vi "MS Operation Thorlabs.vi"(6 "OCT Z PID Gains":cluster{"Kp":dbl, "Kd":dbl, "Ki":dbl}={"Kp"=0.0003, "Kd"=0.0001, "Ki"=0.01}, 8 "error in":errorcluster, 9 "OCT Prev Posit":dbl, 11 "FPGA VI Reference In":refnum<k20>) -> (0 "error out":errorcluster, 1 "OCT Last Posit":dbl, 3 "FPGA VI Reference Out":refnum<k20>)   [LabVIEW 2016]
uses:
  Subsystems/Global Variables.vi
  <vilib>/Platform/TimedLoop/XDataNode/wakeup.ctl
  <vilib>/Platform/TimedLoop/XDataNode/XDNodeRunTimeDep.lvlib
  <vilib>/Platform/TimedLoop/XDataNode/nitl_modes.ctl
  <vilib>/Platform/TimedLoop/XDataNode/timing_clust.ctl
  <vilib>/platform/TimedLoop/XDataNode/XDataNode.xnode
  <vilib>/rvi/interface/nirviReadWriteControl/nirviReadWriteControl.xnode
  Library/KevinLibraryAll/labview/KevLib01.lvlib
  FPGA Bitfiles/PhantomControlPI_FPGATarget_QuadCtr2_E2412E44.lvbitx
  IRISS_FPGA_IO.vi
  NiFpgaLv.dll
  <vilib>/Utility/error.llb/Error Cluster From Error Code.vi
  <vilib>/rvi/errors/niLvFpgaAdjustHostInterfaceError.vi
panel:
  out "Free":dbl[](array[numeric])
  out "Rigid":dbl[](array[numeric])
  out "Hydration On/Off":bool
  out "vac cmd":dbl
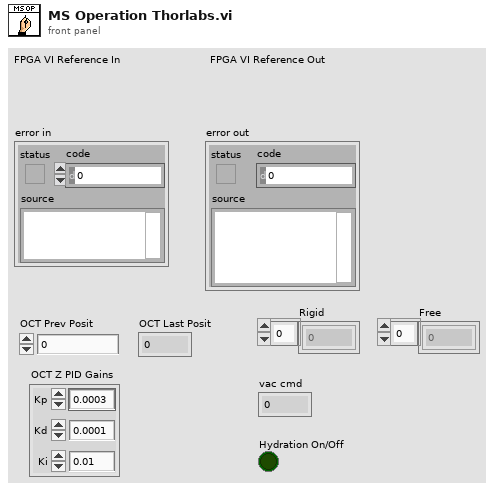
[diagram p1: front panel]
types:
  T1 = typedef "XDNodeRunTimeDep.lvlib/timing_clust.ctl" = cluster{"Expected End [f-1]":u64, "Actual End [f-1]":u64, "Finished Late? [f-1]":bool, "Expected End [i-1]":u64, "Actual End [i-1]":u64, "Finished Late? [i-1]":bool, "Expected Start [i]":u64, "Actual Start [i]":u64, "Expected Start [f]":u64, "Actual Start [f]":u64, "Source Name":string, "Structure Name":string, "Period":i64, "Deadline":i64, "Offset":i64, "Start":i64, "Priority":i32, "Timeout":i32, "Mode":T2, "Wakeup Reason":T3, "Error":errorcluster, "Source Type":string, "Secondary Source Type":string, "Global End Time":u64, "Global Start Time":u64, "Frame Duration":u64, "Iteration Duration":u64, "Assigned CPU":i32, "I/O Scan Engine Mode":u32}
  T2 = typedef "XDNodeRunTimeDep.lvlib/nitl_modes.ctl" = enum32{"No Change", "Process missed periods, maintain original phase", "Discard missed periods, maintain original phase", "Process missed periods, ignore original phase", "Discard missed periods, ignore original phase"}
  T3 = typedef "XDNodeRunTimeDep.lvlib/wakeup.ctl" = enum32{"Normal", "Aborted", "Asynchronous wakeup", "Timing source error", "Timed loop error", "Timeout"}
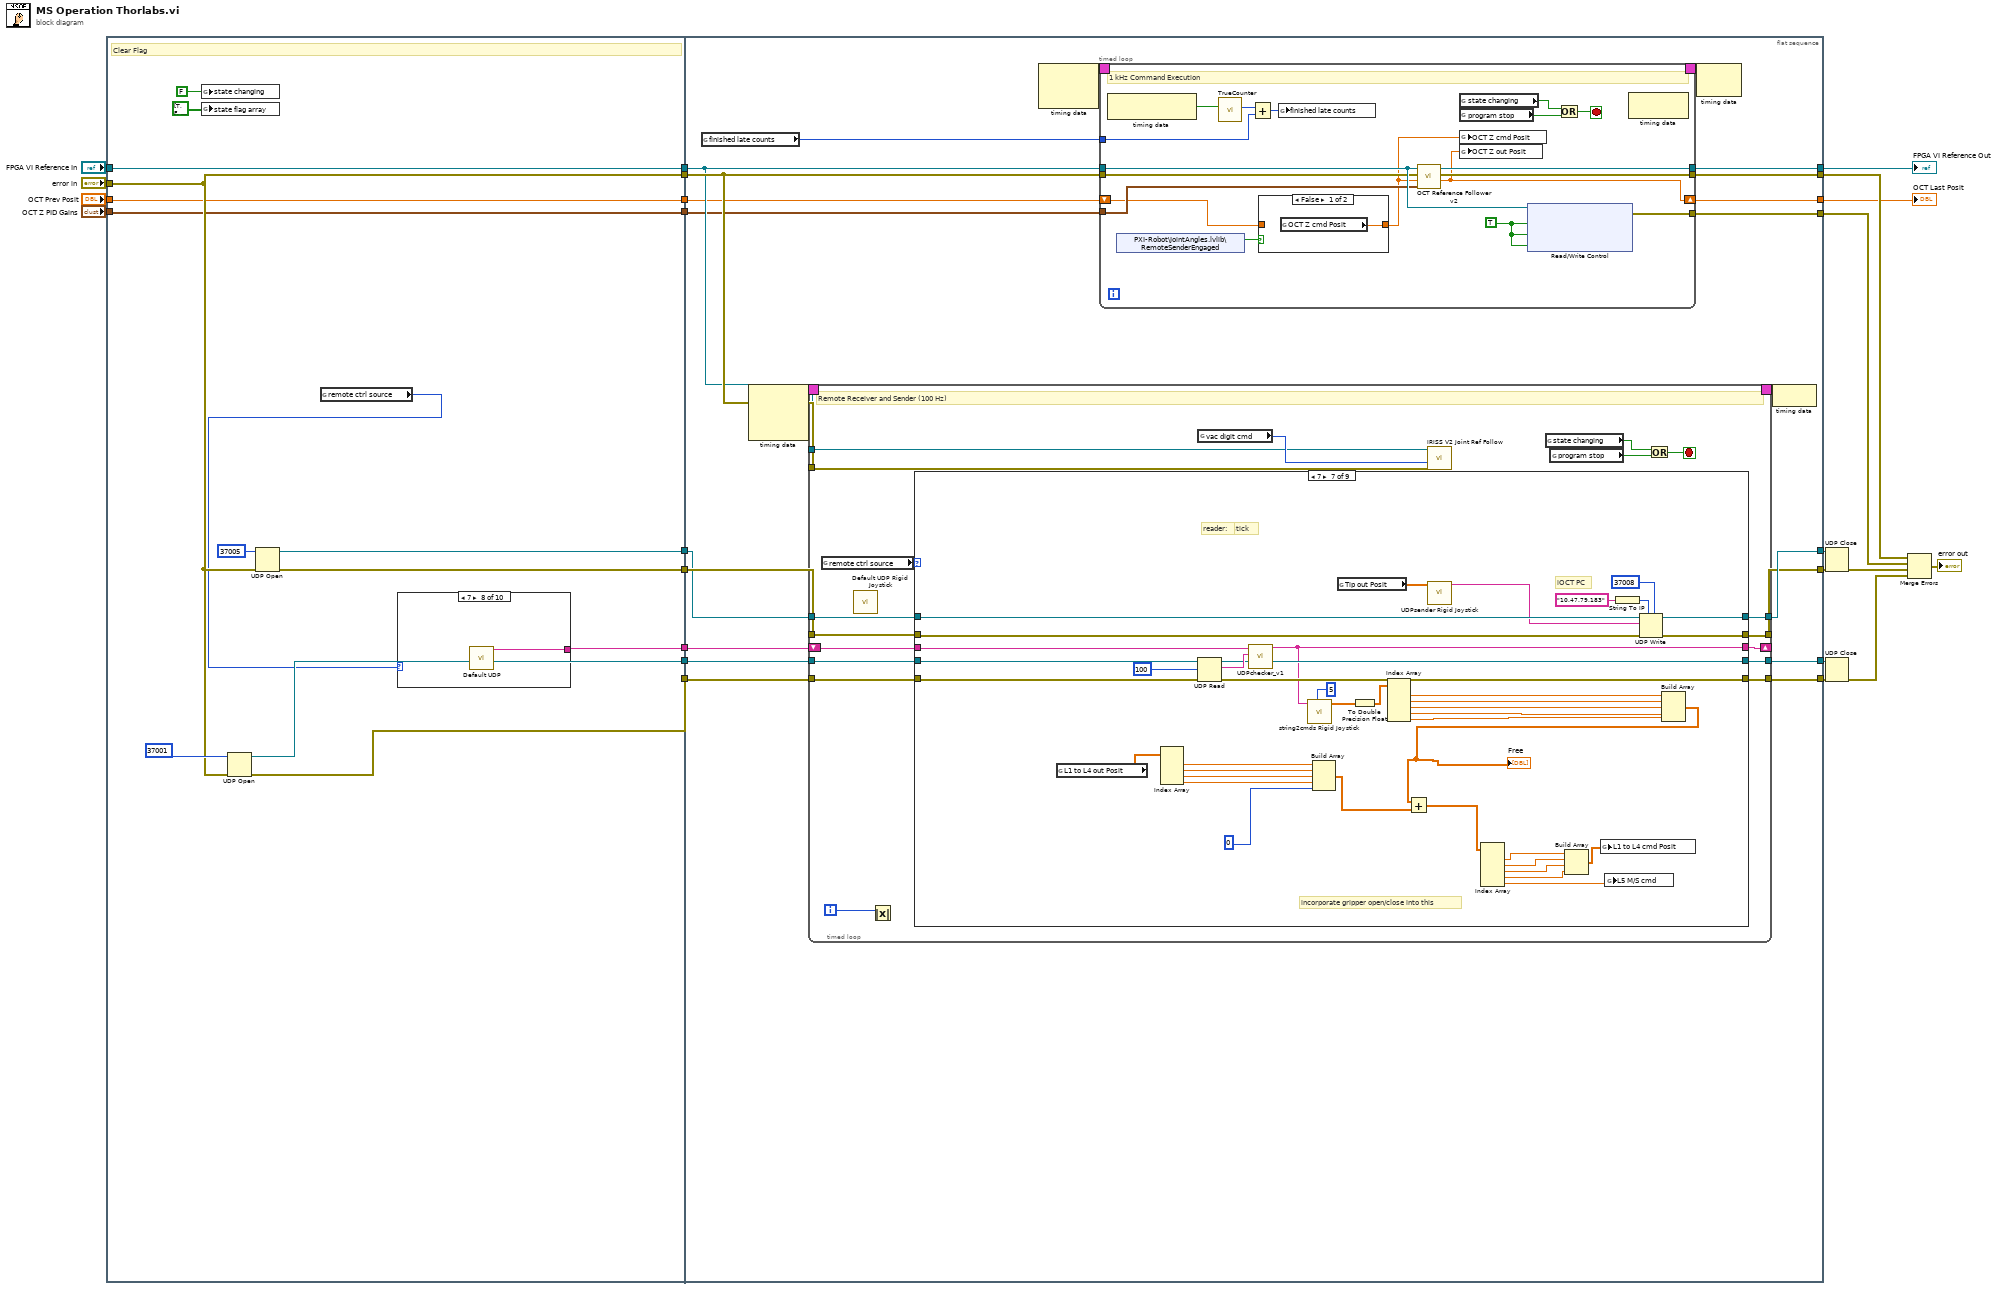
[diagram p0: block diagram]
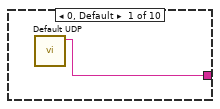
[diagram p2: hidden frame]
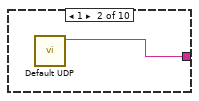
[diagram p3: hidden frame]
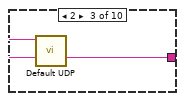
[diagram p4: hidden frame]
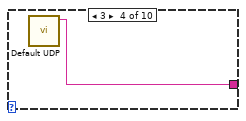
[diagram p5: hidden frame]
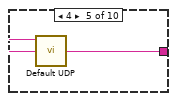
[diagram p6: hidden frame]
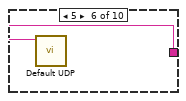
[diagram p7: hidden frame]
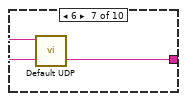
[diagram p8: hidden frame]
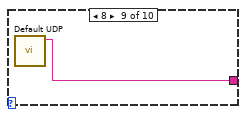
[diagram p9: hidden frame]
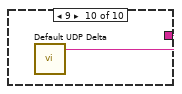
[diagram p10: hidden frame]
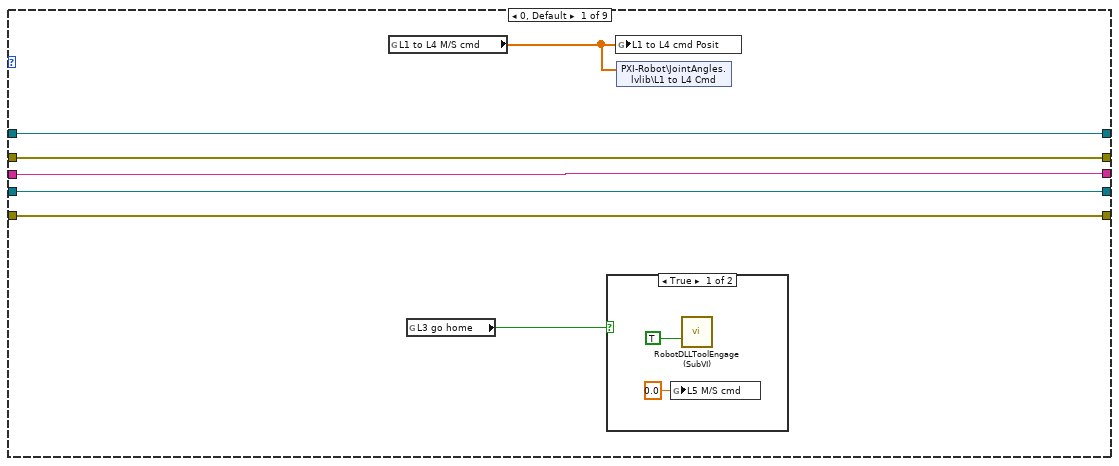
[diagram p11: hidden frame]
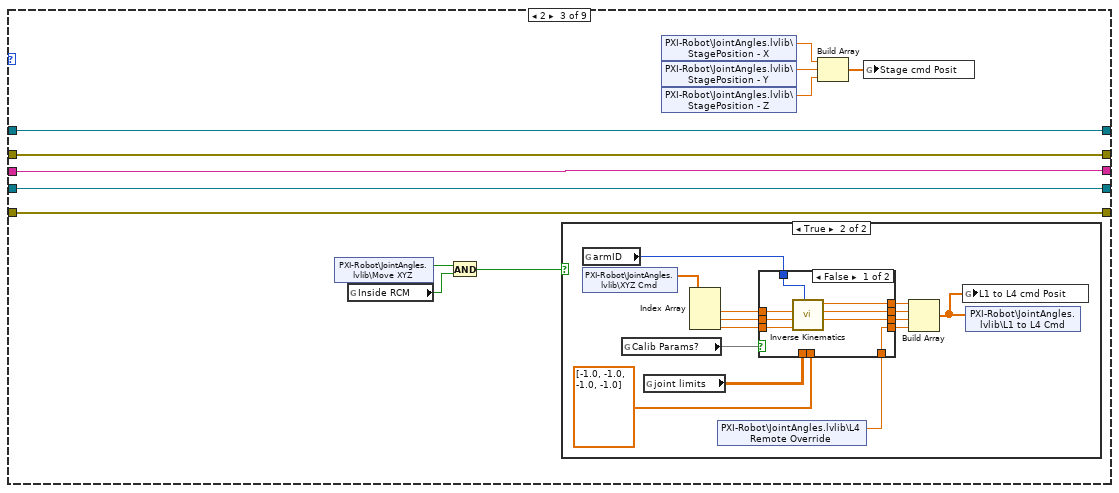
[diagram p14: hidden frame]
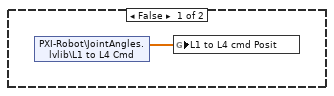
[diagram p15: hidden frame]
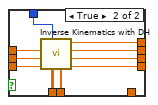
[diagram p16: hidden frame]
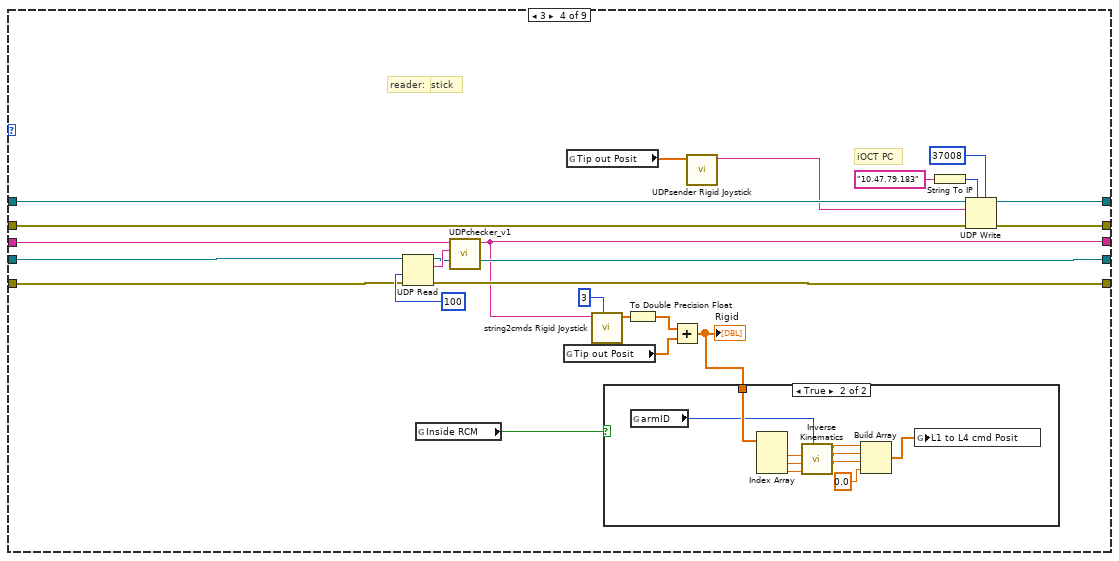
[diagram p17: hidden frame]
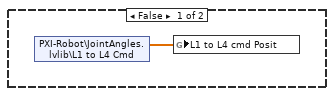
[diagram p18: hidden frame]
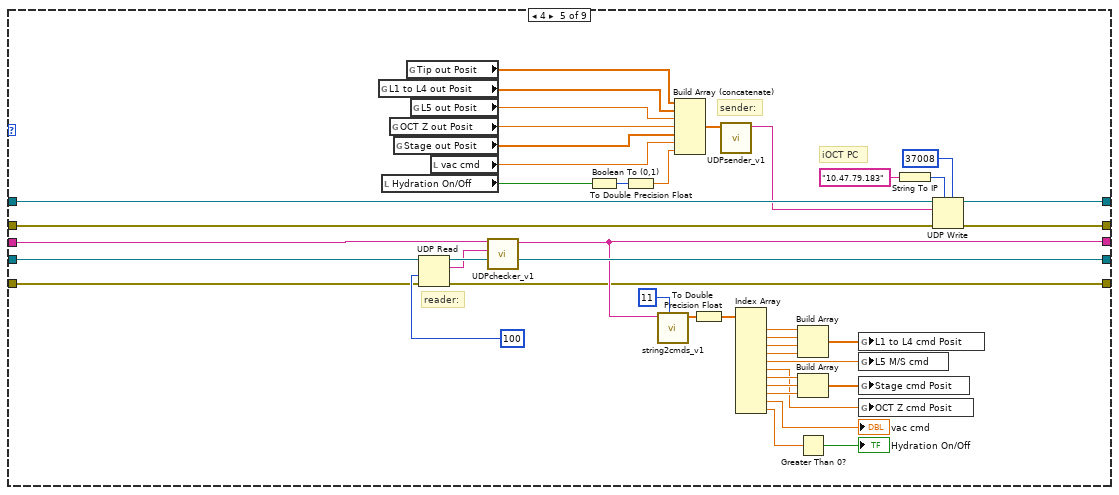
[diagram p19: hidden frame]
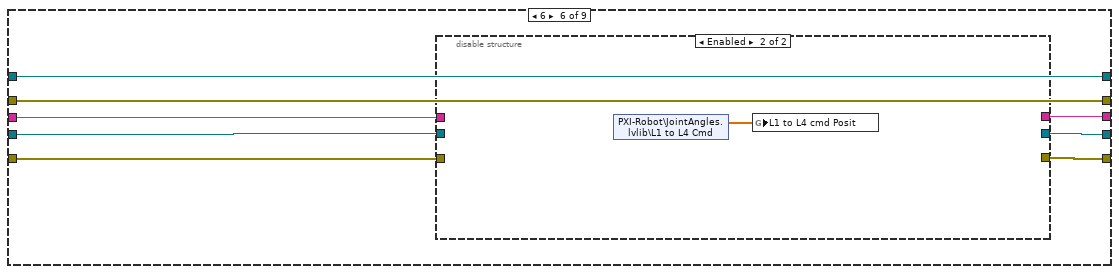
[diagram p20: hidden frame]
diagram:
  n1 = flat-sequence {
    tunnel: [w36] -> w24
    tunnel: "FPGA VI Reference In" -> [w36]
    tunnel: [w28] -> w22
    tunnel: "error in" -> [w28]
    tunnel: [w29] -> w20
    tunnel: [w33] -> w18
    tunnel: [w32] -> w17
    tunnel: [w31] -> w16
    tunnel: [w30] -> w15
    tunnel: [w27] -> w5
    tunnel: "OCT Prev Posit" -> [w27]
    tunnel: [w26] -> w3
    tunnel: "OCT Z PID Gains" -> [w26]
    tunnel: w24 -> [w52]
    tunnel: w22 -> [w53]
    tunnel: [w68] -> w6
    tunnel: [w67] -> w7
    tunnel: [w65] -> w21
    tunnel: w20 -> [w58]
    tunnel: w18 -> [w62]
    tunnel: w17 -> [w61]
    tunnel: w16 -> [w60]
    tunnel: w15 -> [w59]
    tunnel: [w57] -> w12
    tunnel: [w56] -> w11
    tunnel: [w55] -> w10
    tunnel: [w54] -> w9
    tunnel: w5 -> [w51]
    tunnel: w3 -> [w50]
    tunnel: [w49] -> w1
    frame #0 {
      # "Clear Flag"
      n2 = global write "Global Variables.vi" "state changing"(FALSE ("state changing")) -> ()
      n3 = global write "Global Variables.vi" "state flag array"(bool[] [TRUE, FALSE, FALSE, FALSE, FALSE, FALSE, FALSE, FALSE, FALSE] ("state flag array")) -> ()
      n4 = UDP Open(8:w28, 11:u16 37001 ("port")) -> (port=w31:refnum<k16>, 0:w30:errorcluster)  [unwired: 3 in, 1 out]
      n5 = UDP Open(8:w28, 11:u16 37005 ("port")) -> (port=w32:refnum<k16>, 0:w33:errorcluster)  [unwired: 3 in, 1 out]
      n6 = global read "Global Variables.vi" "remote ctrl source"() -> (w25:u16)
      n7 = case shown="7" w25 {
        tunnel: [w39 w40 w41 w42 w43 w44 w45 w46 w47 w48] -> w29
        frame 0, Default {
          n8 = call "Default UDP.vi"() -> ("String"=w39:string)  [unwired: 11 in]
        }
        frame 1 {
          n9 = call "Default UDP.vi"() -> ("String"=w40:string)  [unwired: 11 in]
        }
        frame 2 {
          n10 = call "Default UDP.vi"() -> ("String"=w41:string)  [unwired: 11 in]
        }
        frame 3 {
          n11 = call "Default UDP.vi"() -> ("String"=w42:string)  [unwired: 11 in]
        }
        frame 4 {
          n12 = call "Default UDP.vi"() -> ("String"=w43:string)  [unwired: 11 in]
        }
        frame 5 {
          n13 = call "Default UDP.vi"() -> ("String"=w44:string)  [unwired: 11 in]
        }
        frame 6 {
          n14 = call "Default UDP.vi"() -> ("String"=w45:string)  [unwired: 11 in]
        }
        frame 7 {
          n15 = call "Default UDP.vi"() -> ("String"=w46:string)  [unwired: 11 in]
        }
        frame 8 {
          n16 = call "Default UDP.vi"() -> ("String"=w47:string)  [unwired: 11 in]
        }
        frame 9 {
          n17 = call "Default UDP Delta.vi"() -> ("String"=w48:string)  [unwired: 11 in]
        }
      }
    }
    frame #1 {
      n18 = global read "Global Variables.vi" "finished late counts"() -> (w66:u16)
      n19 = node-c288() -> (w64:T1)  [unwired: 3 in]
      n20 = timed-loop {
        timing: w64 -> [_]
        timing-out: [_] -> w63
        tunnel: w60 -> [w88]
        tunnel: [w87] -> w55
        shift-right: [w85] -> _
        shift-left: w58 -> [w86]
        tunnel: w61 -> [w84]
        tunnel: w62 -> [w83]
        tunnel: [w82] -> w57
        tunnel: [w81] -> w56
        tunnel: w59 -> [w80]
        tunnel: [w79] -> w54
        tunnel: w52 -> [w73]
        tunnel: w53 -> [w72]
        i -> [w71]
        stop <- w76 stop-if-true
        # "Remote Receiver and Sender (100 Hz)"
        n21 = global read "Global Variables.vi" "remote ctrl source"() -> (w75:u16)
        n22 = call "Default UDP Rigid Joystick.vi"() -> ()  [unwired: 11 in, 1 out]
        n23 = Absolute Value(x=w71) -> ()  [unwired: 1 out]
        n24 = case shown="7" w75 {
          tunnel: w88 -> [w92 w99 w111 w168 w223 w229 w287 w292 w318]
          tunnel: [w92 w99 w111 w164 w222 w230 w285 w292 w319] -> w87
          tunnel: w86 -> [w93 w100 w112 w162 w182 w232 w283 w293 w325]
          tunnel: [w93 w100 w112 w161 w209 w231 w282 w293 w314] -> w85
          tunnel: w84 -> [w95 w102 w114 w155 w207 w225 w278 w311 w326]
          tunnel: w83 -> [w94 w101 w113 w153 w206 w226 w276 w310 w324]
          tunnel: [w95 w102 w114 w154 w202 w225 w277 w306 w320] -> w82
          tunnel: [w94 w101 w113 w152 w201 w226 w275 w305 w323] -> w81
          tunnel: w80 -> [w91 w98 w110 w167 w200 w227 w286 w291 w322]
          tunnel: [w91 w98 w110 w163 w199 w228 w284 w291 w321] -> w79
          frame 0, Default {
            n25 = global read "Global Variables.vi" "L1 to L4 M/S cmd"() -> (w89:dbl[])
            n26 = global read "Global Variables.vi" "L3 go home"() -> (w90:bool)
            n27 = case shown="True" w90 {
              frame True {
                n28 = global write "Global Variables.vi" "L5 M/S cmd"(0.0 ("L5 M/S cmd")) -> ()
                n29 = call "RobotDLLToolEngage (SubVI).vi"("Tool Fast Retraction"=TRUE ("Tool Withdraw")) -> ()  [unwired: 18 in, 1 out]
              }
              frame False {
              }
            }
            n30 = global write "Global Variables.vi" "L1 to L4 cmd Posit"(w89) -> ()
            n31 = shared-variable "PXI-Robot\\JointAngles.lvlib\\L1 to L4 Cmd"(w89) -> ()  [unwired: 1 in, 1 out]
          }
          frame 1 {
          }
          frame 2 {
            n32 = shared-variable "PXI-Robot\\JointAngles.lvlib\\Move XYZ"() -> (w108:bool)  [unwired: 1 in, 1 out]
            n33 = global read "Global Variables.vi" "Inside RCM"() -> (w107:bool)
            n34 = And(x=w108, y=w107) -> (x .and. y?=w109:bool)
            n35 = case shown="True" w109 {
              frame False {
                n36 = shared-variable "PXI-Robot\\JointAngles.lvlib\\L1 to L4 Cmd"() -> (w115:dbl[])  [unwired: 1 in, 1 out]
                n37 = global write "Global Variables.vi" "L1 to L4 cmd Posit"(w115) -> ()
              }
              frame True {
                n38 = global read "Global Variables.vi" "armID"() -> (w127:i32)
                n39 = shared-variable "PXI-Robot\\JointAngles.lvlib\\XYZ Cmd"() -> (w129:dbl[])  [unwired: 1 in, 1 out]
                n40 = global read "Global Variables.vi" "Calib Params?"() -> (w116)
                n41 = global read "Global Variables.vi" "joint limits"() -> (w119:dbl[][])
                n42 = Index Array(array=w129) -> (element #1=w126:dbl, element #2=w125:dbl, element #3=w124:dbl)  [unwired: 3 in]
                n43 = shared-variable "PXI-Robot\\JointAngles.lvlib\\L4 Remote Override"() -> (w117:dbl)  [unwired: 1 in, 1 out]
                n44 = case shown="False" w116 {
                  tunnel: w127 -> [w130 w147]
                  tunnel: w126 -> [w137 w146]
                  tunnel: w125 -> [w136 w145]
                  tunnel: w124 -> [w135 w144]
                  tunnel: [w134 w143] -> w123
                  tunnel: [w133 w142] -> w122
                  tunnel: [w132 w141] -> w121
                  tunnel: dbl[] [-1.0, -1.0, -1.0, -1.0] ("Initial guess") -> [_ w140]
                  tunnel: w119 -> [_ w139]
                  tunnel: [w131 w138] -> w118
                  tunnel: w117 -> [w131 _]
                  frame False {
                    n45 = call "Inverse Kinematics.vi"("armID"=w130, "z"=w135, "y"=w136, "x"=w137) -> ("j3"=w132:dbl, "j2"=w133:dbl, "j1"=w134:dbl)  [unwired: 4 in, 1 out]
                  }
                  frame True {
                    n46 = call "Inverse Kinematics with DH.vi"("Initial guess"=w140, "Joint Limits"=w139, "armID"=w147, "z"=w144, "y"=w145, "x"=w146) -> ("j4"=w138:dbl, "j3"=w141:dbl, "j2"=w142:dbl, "j1"=w143:dbl)  [unwired: 2 in]
                  }
                }
                n47 = Build Array(w123, w122, w121, w118) -> (w128:dbl[])
                n48 = global write "Global Variables.vi" "L1 to L4 cmd Posit"(w128) -> ()
                n49 = shared-variable "PXI-Robot\\JointAngles.lvlib\\L1 to L4 Cmd"(w128) -> ()  [unwired: 1 in, 1 out]
              }
            }
            n50 = shared-variable "PXI-Robot\\JointAngles.lvlib\\StagePosition - X"() -> (w106:dbl)  [unwired: 1 in, 1 out]
            n51 = shared-variable "PXI-Robot\\JointAngles.lvlib\\StagePosition - Y"() -> (w105:dbl)  [unwired: 1 in, 1 out]
            n52 = shared-variable "PXI-Robot\\JointAngles.lvlib\\StagePosition - Z"() -> (w104:dbl)  [unwired: 1 in, 1 out]
            n53 = Build Array(w106, w105, w104) -> (w103:dbl[])
            n54 = global write "Global Variables.vi" "Stage cmd Posit"(w103) -> ()
          }
          frame 3 {
            # "Rigid Joystick"
            # "iOCT PC"
            # "reader:"
            n55 = UDP Read(connection ID=w168, timeout ms (25000)=100, 8:w167) -> (data out=w169:string, error out=w163:errorcluster, 3:w164:refnum<k16>)  [unwired: 1 in, 2 out]
            n56 = global read "Global Variables.vi" "Inside RCM"() -> (w166:bool)
            n57 = call "UDPchecker_v1.vi"("new string"=w169, "old string"=w162) -> ("output string"=w161:string)  [unwired: 9 in]
            n58 = global read "Global Variables.vi" "Tip out Posit"() -> (w158:dbl[])
            n59 = global read "Global Variables.vi" "Tip out Posit"() -> (w149:dbl[])
            n60 = call "string2cmds Rigid Joystick.vi"("numCmds"=3, "input string"=w161) -> ("output cmds"=w160:dbl[])  [unwired: 9 in]
            n61 = To Double Precision Float(number=w160) -> (double precision float=w165:dbl[])
            n62 = Add(x=w165, y=w158) -> (x+y=w157:dbl[])
            "Rigid" <- w157
            n63 = case shown="True" w166 {
              tunnel: w157 -> [_ w179]
              frame False {
                n64 = shared-variable "PXI-Robot\\JointAngles.lvlib\\L1 to L4 Cmd"() -> (w171:dbl[])  [unwired: 1 in, 1 out]
                n65 = global write "Global Variables.vi" "L1 to L4 cmd Posit"(w171) -> ()
              }
              frame True {
                n66 = global read "Global Variables.vi" "armID"() -> (w175:i32)
                n67 = Index Array(array=w179) -> (element #1=w178:dbl, element #2=w177:dbl, element #3=w176:dbl)  [unwired: 3 in]
                n68 = call "Inverse Kinematics.vi"("armID"=w175, "z"=w176, "y"=w177, "x"=w178) -> ("j3"=w172:dbl, "j2"=w173:dbl, "j1"=w174:dbl)  [unwired: 4 in, 1 out]
                n69 = Build Array(w174, w173, w172, 0.0 ("element")) -> (w181:dbl[])
                n70 = global write "Global Variables.vi" "L1 to L4 cmd Posit"(w181) -> ()
              }
            }
            n71 = call "UDPsender Rigid Joystick.vi"("nums2send"=w149) -> ("string2send"=w150:string)  [unwired: 10 in]
            n72 = String To IP(1:"10.47.79.183" ("name")) -> (0:w151:u32)
            n73 = UDP Write(address=w151, port or service name=u16 37008, connection ID=w155, data in=w150, 8:w153) -> (error out=w152:errorcluster, 3:w154:refnum<k16>)  [unwired: 1 in]
          }
          frame 4 {
            # "sender:"
            # "reader:"
            # "iOCT PC"
            n74 = global read "Global Variables.vi" "L1 to L4 out Posit"() -> (w192:dbl[])
            n75 = local read "Hydration On/Off"() -> (w195:bool)
            n76 = global read "Global Variables.vi" "OCT Z out Posit"() -> (w190:dbl)
            n77 = global read "Global Variables.vi" "Stage out Posit"() -> (w189:dbl[])
            n78 = global read "Global Variables.vi" "Tip out Posit"() -> (w183:dbl[])
            n79 = global read "Global Variables.vi" "L5 out Posit"() -> (w191:dbl)
            n80 = UDP Read(connection ID=w223, timeout ms (25000)=100, 8:w200) -> (data out=w208:string, error out=w199:errorcluster, 3:w222:refnum<k16>)  [unwired: 1 in, 2 out]
            n81 = local read "vac cmd"() -> (w196:dbl)
            n82 = call "UDPchecker_v1.vi"("new string"=w208, "old string"=w182) -> ("output string"=w209:string)  [unwired: 9 in]
            n83 = Boolean To (0,1)(Boolean=w195) -> (0, 1=w194:i16)
            n84 = To Double Precision Float(number=w194) -> (double precision float=w193:dbl)
            n85 = call "string2cmds_v1.vi"("numCmds"=11, "input string"=w209) -> ("output cmds"=w214:sgl[])  [unwired: 9 in]
            n86 = Build Array (concatenate)(w183, w192, w191, w190, w189, w196, w193) -> (w197:dbl[])
            n87 = To Double Precision Float(number=w214) -> (double precision float=w213:dbl[])
            n88 = call "UDPsender_v1.vi"("nums2send"=w197) -> ("string2send"=w198:string)  [unwired: 10 in]
            n89 = Index Array(array=w213) -> (element #1=w220:dbl, element #2=w219:dbl, element #3=w218:dbl, element #4=w185:dbl, element #5=w184:dbl, element #6=w187:dbl, element #7=w217:dbl, element #8=w216:dbl, element #9=w215:dbl, element #10=→"vac cmd":dbl, element #11=w211:dbl)  [unwired: 11 in]
            n90 = Build Array(w220, w219, w218, w185) -> (w186:dbl[])
            n91 = Build Array(w217, w216, w215) -> (w188:dbl[])
            n92 = Greater Than 0?(x=w211) -> (x > 0?=→"Hydration On/Off":bool)
            n93 = global write "Global Variables.vi" "L1 to L4 cmd Posit"(w186) -> ()
            n94 = global write "Global Variables.vi" "L5 M/S cmd"(w184) -> ()
            n95 = global write "Global Variables.vi" "Stage cmd Posit"(w188) -> ()
            n96 = global write "Global Variables.vi" "OCT Z cmd Posit"(w187) -> ()
            n97 = String To IP(1:"10.47.79.183" ("name")) -> (0:w204:u32)
            n98 = UDP Write(address=w204, port or service name=u16 37008, connection ID=w207, data in=w198, 8:w206) -> (error out=w201:errorcluster, 3:w202:refnum<k16>)  [unwired: 1 in]
          }
          frame 6 {
            n99 = disable-structure shown="Enabled" {
              disable-tunnel: w232 -> [w238 _]
              disable-tunnel: [w237 _] -> w231
              disable-tunnel: [w236 _] -> w230
              disable-tunnel: w229 -> [w235 _]
              disable-tunnel: [w234 _] -> w228
              disable-tunnel: w227 -> [w233 _]
              frame Disabled {
                # "reader:"
                n100 = UDP Read(connection ID=w235, timeout ms (25000)=100, 8:w233) -> (data out=w246:string, error out=w234:errorcluster, 3:w236:refnum<k16>)  [unwired: 1 in, 2 out]
                n101 = call "UDPchecker_v1.vi"("new string"=w246, "old string"=w238) -> ("output string"=w237:string)  [unwired: 9 in]
                n102 = call "string2cmds_v1.vi"("numCmds"=4, "input string"=w237) -> ("output cmds"=w244:sgl[])  [unwired: 9 in]
                n103 = To Double Precision Float(number=w244) -> (double precision float=w245:dbl[])
                n104 = Index Array(array=w245) -> (element #1=w241:dbl, element #2=w242:dbl, element #3=w243:dbl, element #4=w248:dbl)  [unwired: 4 in]
                n105 = Build Array(w241, w242, w243, w248) -> (w247:dbl[])
                n106 = global write "Global Variables.vi" "L1 to L4 cmd Posit"(w247) -> ()
              }
              frame Enabled {
                n107 = shared-variable "PXI-Robot\\JointAngles.lvlib\\L1 to L4 Cmd"() -> (w249:dbl[])  [unwired: 1 in, 1 out]
                n108 = global write "Global Variables.vi" "L1 to L4 cmd Posit"(w249) -> ()
              }
            }
          }
          frame 7 {
            # "incorporate gripper open/close into this"
            # "Rigid Joystick"
            # "iOCT PC"
            # "reader:"
            n109 = global read "Global Variables.vi" "L1 to L4 out Posit"() -> (w266:dbl[])
            n110 = Index Array(array=w266) -> (element #1=w265:dbl, element #2=w264:dbl, element #3=w263:dbl, element #4=w254:dbl)  [unwired: 4 in]
            n111 = UDP Read(connection ID=w287, timeout ms (25000)=100, 8:w286) -> (data out=w288:string, error out=w284:errorcluster, 3:w285:refnum<k16>)  [unwired: 1 in, 2 out]
            n112 = call "UDPchecker_v1.vi"("new string"=w288, "old string"=w283) -> ("output string"=w282:string)  [unwired: 9 in]
            n113 = call "string2cmds Rigid Joystick.vi"("numCmds"=5, "input string"=w282) -> ("output cmds"=w281:dbl[])  [unwired: 9 in]
            n114 = Build Array(w265, w264, w263, w254, 0) -> (w251:dbl[])
            n115 = global read "Global Variables.vi" "Tip out Posit"() -> (w272:dbl[])
            n116 = To Double Precision Float(number=w281) -> (double precision float=w270:dbl[])
            n117 = Index Array(array=w270) -> (element #1=w268:dbl, element #2=w269:dbl, element #3=w267:dbl, element #4=w256:dbl, element #5=w255:dbl)  [unwired: 5 in]
            n118 = call "UDPsender Rigid Joystick.vi"("nums2send"=w272) -> ("string2send"=w273:string)  [unwired: 10 in]
            n119 = String To IP(1:"10.47.79.183" ("name")) -> (0:w274:u32)
            n120 = UDP Write(address=w274, port or service name=u16 37008, connection ID=w278, data in=w273, 8:w276) -> (error out=w275:errorcluster, 3:w277:refnum<k16>)  [unwired: 1 in]
            n121 = Build Array(w268, w269, w267, w256, w255) -> (w252:dbl[])
            "Free" <- w252
            n122 = Add(x=w252, y=w251) -> (x+y=w250:dbl[])
            n123 = Index Array(array=w250) -> (element #1=w261:dbl, element #2=w260:dbl, element #3=w259:dbl, element #4=w257:dbl, element #5=w258:dbl)  [unwired: 5 in]
            n124 = Build Array(w261, w260, w259, w257) -> (w262:dbl[])
            n125 = global write "Global Variables.vi" "L1 to L4 cmd Posit"(w262) -> ()
            n126 = global write "Global Variables.vi" "L5 M/S cmd"(w258) -> ()
          }
          frame 8 {
            # "Zeiss PC"
            # "sender:"
            # "iOCT PC"
            n127 = global read "Global Variables.vi" "L1 to L4 out Posit"() -> (w299:dbl[])
            n128 = local read "Hydration On/Off"() -> (w290:bool)
            n129 = global read "Global Variables.vi" "L1 to L4 M/S cmd"() -> (w294:dbl[])
            n130 = global read "Global Variables.vi" "OCT Z out Posit"() -> (w297:dbl)
            n131 = global read "Global Variables.vi" "Stage out Posit"() -> (w296:dbl[])
            n132 = global read "Global Variables.vi" "Tip out Posit"() -> (w295:dbl[])
            n133 = global read "Global Variables.vi" "L5 out Posit"() -> (w298:dbl)
            n134 = local read "vac cmd"() -> (w302:dbl)
            n135 = Boolean To (0,1)(Boolean=w290) -> (0, 1=w301:i16)
            n136 = global write "Global Variables.vi" "L1 to L4 cmd Posit"(w294) -> ()
            n137 = shared-variable "PXI-Robot\\JointAngles.lvlib\\L1 to L4 Cmd"(w294) -> ()  [unwired: 1 in, 1 out]
            n138 = To Double Precision Float(number=w301) -> (double precision float=w300:dbl)
            n139 = Build Array (concatenate)(w295, w299, w298, w297, w296, w302, w300) -> (w303:dbl[])
            n140 = call "UDPsender_v1.vi"("nums2send"=w303) -> ("string2send"=w304:string)  [unwired: 10 in]
            n141 = String To IP(1:"10.47.79.183" ("name")) -> (0:w308:u32)
            n142 = UDP Write(address=w308, port or service name=u16 37008, connection ID=w311, data in=w304, 8:w310) -> (error out=w305:errorcluster, 3:w306:refnum<k16>)  [unwired: 1 in]
          }
          frame 9 {
            # "Zeiss PC"
            # "Add delta commands to current joint angles"
            # "sender:"
            # "reader:"
            # "iOCT PC"
            n143 = global read "Global Variables.vi" "L1 to L4 out Posit"() -> (w332:dbl[])
            n144 = local read "Hydration On/Off"() -> (w335:bool)
            n145 = global read "Global Variables.vi" "OCT Z out Posit"() -> (w330:dbl)
            n146 = global read "Global Variables.vi" "Stage out Posit"() -> (w329:dbl[])
            n147 = global read "Global Variables.vi" "Tip out Posit"() -> (w327:dbl[])
            n148 = global read "Global Variables.vi" "L5 out Posit"() -> (w331:dbl)
            n149 = UDP Read(connection ID=w318, timeout ms (25000)=100, 8:w322) -> (data out=w342:string, error out=w321:errorcluster, 3:w319:refnum<k16>)  [unwired: 1 in, 2 out]
            n150 = local read "vac cmd"() -> (w336:dbl)
            n151 = call "UDPchecker_v1.vi"("new string"=w342, "old string"=w325) -> ("output string"=w314:string)  [unwired: 9 in]
            n152 = global read "Global Variables.vi" "L1 to L4 out Posit"() -> (w316:dbl[])
            n153 = Boolean To (0,1)(Boolean=w335) -> (0, 1=w334:i16)
            n154 = To Double Precision Float(number=w334) -> (double precision float=w333:dbl)
            n155 = call "string2cmds Rigid Joystick.vi"("numCmds"=4, "input string"=w314) -> ("output cmds"=w312:dbl[])  [unwired: 9 in]
            n156 = Build Array (concatenate)(w327, w332, w331, w330, w329, w336, w333) -> (w337:dbl[])
            n157 = To Double Precision Float(number=w312) -> (double precision float=w343:dbl[])
            n158 = call "UDPsender_v1.vi"("nums2send"=w337) -> ("string2send"=w338:string)  [unwired: 10 in]
            n159 = Index Array(array=w343) -> (element #1=w346:dbl, element #2=w345:dbl, element #3=w344:dbl, element #4=w328:dbl)  [unwired: 4 in]
            n160 = Build Array(w346, w345, w344, w328) -> (w317:dbl[])
            n161 = Add(x=w317, y=w316) -> (x+y=w315:dbl[])
            n162 = String To IP(1:"10.47.79.183" ("name")) -> (0:w340:u32)
            n163 = UDP Write(address=w340, port or service name=u16 37008, connection ID=w326, data in=w338, 8:w324) -> (error out=w323:errorcluster, 3:w320:refnum<k16>)  [unwired: 1 in]
            n164 = global write "Global Variables.vi" "L1 to L4 cmd Posit"(w315) -> ()
          }
        }
        n165 = global read "Global Variables.vi" "vac digit cmd"() -> (w74:i8)
        n166 = call "IRISS V2 Joint Ref Follow.vi"("error in"=w72, "Digital Cmd [0-78]"=w74, "FPGA VI Reference In"=w73) -> ()  [unwired: 5 in, 2 out]
        n167 = global read "Global Variables.vi" "state changing"() -> (w78:bool)
        n168 = global read "Global Variables.vi" "program stop"() -> (w77:bool)
        n169 = Or(x=w78, y=w77) -> (x .or. y?=w76:bool)
      }
      n170 = node-c288() -> (w70:T1)  [unwired: 2 in]
      n171 = timed-loop {
        timing: w70 -> [_]
        timing-out: [_] -> w69
        tunnel: w52 -> [w361]
        tunnel: w53 -> [w359]
        tunnel: [w367] -> w68
        tunnel: [w360] -> w65
        tunnel: [w358] -> w67
        tunnel: w66 -> [w356]
        tunnel: w50 -> [w357]
        shift-right: [w352] -> w49
        shift-left: w51 -> [w354]
        stop <- w369 stop-if-true
        w362 = TRUE ("Conn0/DIO15 Button 4")
        # "1 kHz Command Execution"
        n172 = node-c288() -> (w365:bool)  [unwired: 1 in]
        n173 = shared-variable "PXI-Robot\\JointAngles.lvlib\\RemoteSenderEngaged"() -> (w355:bool)  [unwired: 1 in, 1 out]
        n174 = call "TrueCounter.vi"("True?"=w365) -> ("True Count"=w363:u16)  [unwired: 10 in]
        n175 = Add(x=w363, y=w356) -> (x+y=w364:u16)
        n176 = case shown="False" w355 {
          tunnel: [w370 w371] -> w353
          tunnel: w354 -> [_ _]
          frame False {
            n177 = global read "Global Variables.vi" "OCT Z cmd Posit"() -> (w370:dbl)
          }
          frame True {
            n178 = shared-variable "PXI-Robot\\JointAngles.lvlib\\OCT z command"() -> (w371:dbl)  [unwired: 1 in, 1 out]
          }
        }
        n179 = global write "Global Variables.vi" "finished late counts"(w364) -> ()
        n180 = call "OCT Reference Follower v2.vi"("OCT Z PID Gains"=w357, "OCT  Z cmd Posit [mm]"=w353, "error in"=w359, "FPGA VI Reference In"=w361) -> ("OCT  Z out Posit [mm]"=w352:dbl, "error out"=w358:errorcluster, "FPGA VI Reference Out"=w360:refnum<k20>)  [unwired: 5 in]
        n181 = global read "Global Variables.vi" "state changing"() -> (w368:bool)
        n182 = global read "Global Variables.vi" "program stop"() -> (w366:bool)
        n183 = global write "Global Variables.vi" "OCT Z cmd Posit"(w353) -> ()
        n184 = global write "Global Variables.vi" "OCT Z out Posit"(w352) -> ()
        n185 = xnode "Read/Write Control"("FPGA VI Reference In"=w361, "Conn0/DIO12 Button 1"=w362, "Conn0/DIO13 Button 2"=w362, "Conn0/DIO15 Button 4"=w362) -> ("error out"=w367:errorcluster)  [unwired: 1 in, 1 out]
        n186 = Or(x=w368, y=w366) -> (x .or. y?=w369:bool)
        n187 = node-c288() -> ()  [unwired: 1 in, 1 out]
      }
      n188 = node-c288(w69) -> ()  [unwired: 1 out]
      n189 = node-c288(w63) -> ()
    }
  }
  n190 = UDP Close(connection ID=w12, 8:w11) -> (error out=w13:errorcluster)  [unwired: 1 out]
  n191 = UDP Close(connection ID=w10, 8:w9) -> (error out=w14:errorcluster)  [unwired: 1 out]
  n192 = Merge Errors(w7, w6, w13, w14) -> (→"error out":errorcluster)
  "FPGA VI Reference Out" <- w21
  "OCT Last Posit" <- w1
